vi "_Obtain Promise.vi"(8 "error in (no error)":errorcluster, 9 "create if not found? (T)":bool, 10 "name (unnamed)":string, 11 "Future in":refnum<class "Promise.lvclass">) -> (0 "error out":errorcluster, 2 "created new?":bool, 3 "Future out":refnum<class "Promise.lvclass">)   [LabVIEW 2017, in "Promise.lvlib" / "Promise.lvclass"]
uses:
  Promise.lvclass
  Promise.lvclass/Promise.ctl
  <vilib>/Utility/error.llb/Error Cluster From Error Code.vi
  <vilib>/ErrorRing/Error Ring.xnode
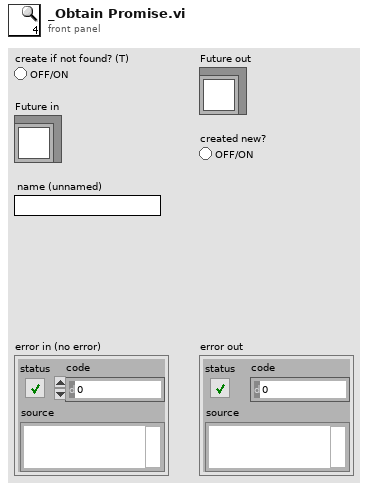
[diagram p1: front panel]
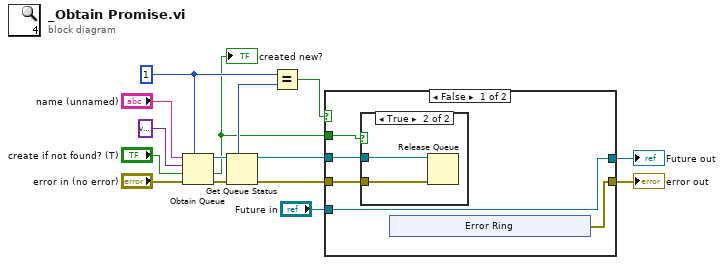
[diagram p0: block diagram]
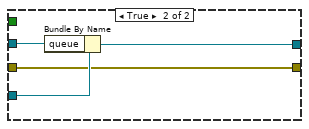
[diagram p3: hidden frame]
diagram:
  w15 = 1 ("max queue size (-1, unlimited)")
  n1 = Obtain Queue(max queue size (-1, unlimited)=w15, name (unnamed)="name (unnamed)", element data type=variant, create if not found? (T)="create if not found? (T)", error in (no error)="error in (no error)") -> (queue out=w10:refnum<queue>, created new?=w1:bool, error out=w9:errorcluster)
  "created new?" <- w1
  n2 = Get Queue Status(queue=w10, error in (no error)=w9) -> (queue out=w11:refnum<queue>, max queue size=w14:i32, error out=w13:errorcluster)  [unwired: 1 in, 5 out]
  n3 = Equal?(x=w15, y=w14) -> (x = y?=w12:bool)
  n4 = case shown="False" w12 {
    tunnel: [w20 w28] -> w3
    tunnel: "Future in" -> [w19 w31]
    tunnel: [w19 w30] -> w5
    tunnel: w11 -> [w17 w29]
    tunnel: w13 -> [w16 w28]
    tunnel: w1 -> [w18 _]
    frame False {
      n5 = case shown="True" w18 {
        tunnel: w17 -> [_ w22]
        tunnel: w16 -> [_ w21]
        frame False {
        }
        frame True {
          n6 = Release Queue(queue=w22, error in (no error)=w21) -> ()  [unwired: 1 in, 3 out]
        }
      }
      n7 = xnode "Error Ring"() -> ("error out"=w20:errorcluster)
    }
    frame True {
      n8 = Bundle By Name(cluster=w31, "queue"=w29) -> (w30:refnum<class "Promise.lvclass">)
    }
  }
  "Future out" <- w5
  "error out" <- w3
